vi "HEWH Check Reset Condition.vi"(8 "Error In":errorcluster, 10 "SC3 Check Skip":T1, 11 "Current Cond":T1) -> (0 "Error Out":errorcluster, 2 "Equals Reset Fail?":bool, 3 "Current Cond":T1)   [LabVIEW 2016]
uses:
  Type Definitions/HEWH Special Condition Check.ctl
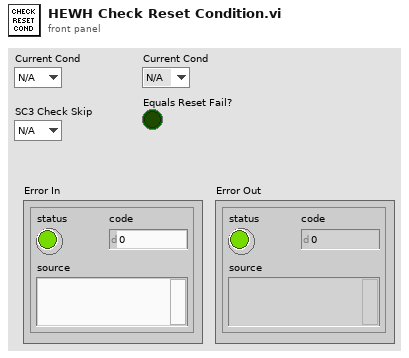
[diagram p1: front panel]
types:
  T1 = typedef "HEWH Special Condition Check.ctl" = enum16{"N/A", "C1", "C2", "Reset/Fail", "Skip Draw Sequence"}
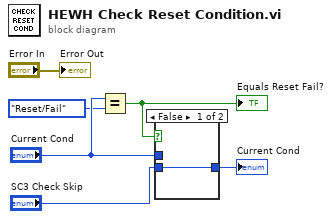
[diagram p0: block diagram]
diagram:
  n1 = Equal?(x="Current Cond", y=HEWH_Special_Condition_Check."Reset/Fail") -> (x = y?=w3:bool)
  "Equals Reset Fail?" <- w3
  n2 = case shown="False" w3 {
    tunnel: "Current Cond" -> [_ w8]
    tunnel: [w7 w8] -> w6
    tunnel: "SC3 Check Skip" -> [w7 _]
    frame False {
    }
    frame True {
    }
  }
  "Current Cond" <- w6
  "Error Out" <- "Error In"
